vi "FPGA_ADSRFilter.vi"(11 "ADSR Settings":T1) -> ()   [LabVIEW 2014]
uses:
  Desktop/Envelope Filter/ADSR State.ctl
  <vilib>/rvi/FXPMathLib/FxpDiv/subVIs/nifxpmath_Div_SimConfig.ctl
  <vilib>/rvi/Emulation/niFpgaGetClockAttributes.vi
  <vilib>/rvi/Emulation/niFpgaSctlEmulationGetInTimedLoop.vi
  <vilib>/rvi/Emulation/niFpgaEmulationReportErrorSimple.vi
  <vilib>/rvi/FXPMathLib/FxpDiv/simVIs/DllFxpDivTemp_sub.vi
  <vilib>/rvi/Emulation/niFpgaCriticalErrorInLSC.vi
  MIDI/Controls/Stop.vi
  <vilib>/rvi/FXPMathLib/FxpDiv/XNode/nifxpmath_Div.xnode
  <vilib>/rvi/FXPMathLib/FxpMul/XNode/nifxpmath_Multiplier.xnode
  <vilib>/rvi/FXPMathLib/FxpSub/XNode/nifxpmath_Sub.xnode
  <vilib>/rvi/FXPMathLib/sim/FxpSim.dll
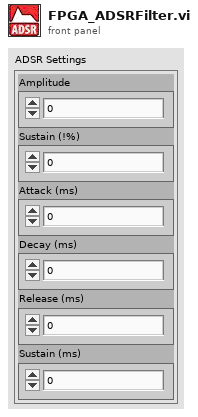
[diagram p1: front panel]
types:
  T1 = cluster{"Amplitude":fxp<+,10,1>, "Sustain (!%) ":fxp<+,10,1>, "Attack (ms)":fxp<+,11,11>, "Decay (ms) ":fxp<+,11,11>, "Release (ms)":fxp<+,11,11>, "Sustain (ms)":fxp<+,11,11>}
  T2 = typedef "ADSR State.ctl" = enum16{"Attack", "Decay", "Sustain", "Release"}
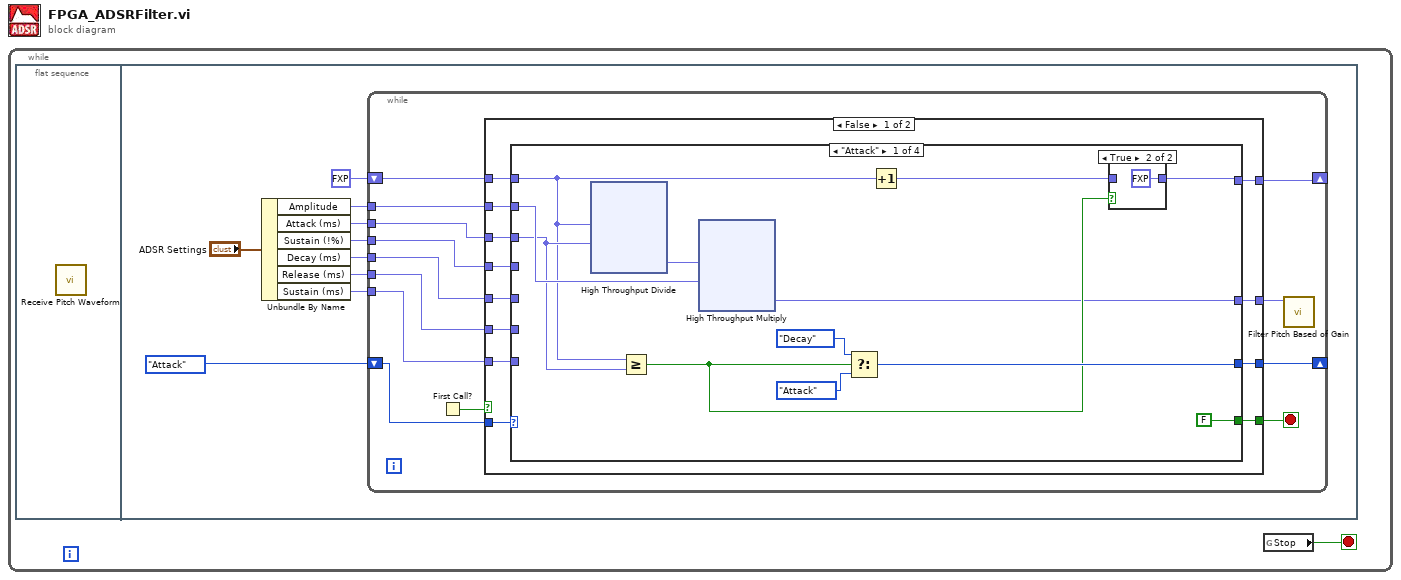
[diagram p0: block diagram]
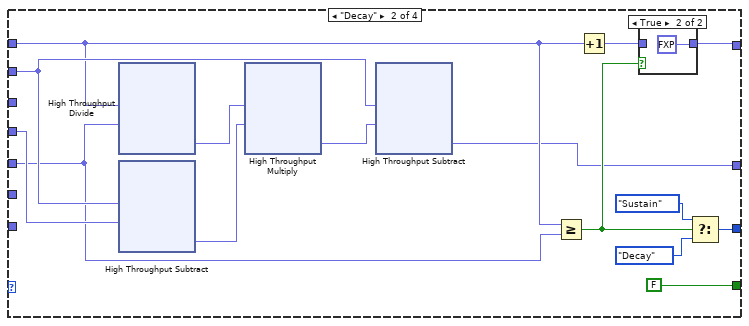
[diagram p3: hidden frame]
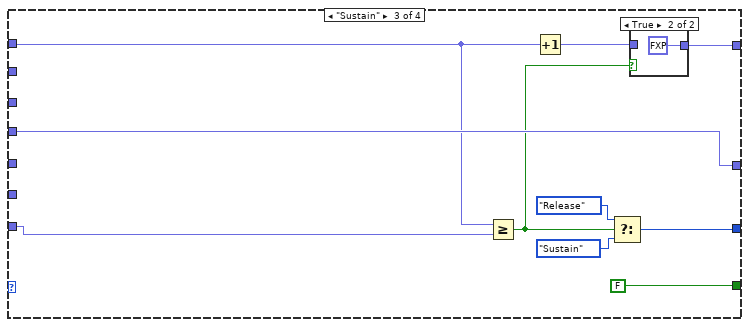
[diagram p5: hidden frame]
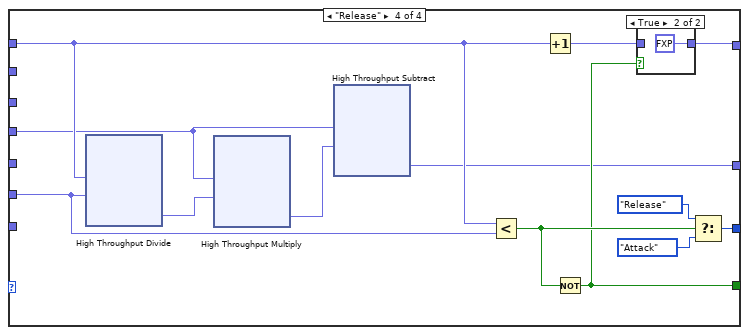
[diagram p7: hidden frame]
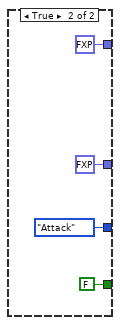
[diagram p9: hidden frame]
diagram:
  n1 = while {
    stop <- w1 stop-if-true
    n2 = flat-sequence {
      frame #0 {
        n3 = call "Receive Pitch Waveform.vi"() -> ()  [unwired: 12 in]
      }
      frame #1 {
        n4 = Unbundle By Name("ADSR Settings") -> ("Amplitude"=w7:fxp<+,10,1>, "Attack (ms)"=w6:fxp<+,11,11>, "Sustain (!%)"=w5:fxp<+,10,1>, "Decay (ms)"=w4:fxp<+,11,11>, "Release (ms)"=w3:fxp<+,11,11>, "Sustain (ms)"=w2:fxp<+,11,11>)
        n5 = while {
          shift-right: [w22] -> _
          shift-left: ADSR_State."Attack" -> [w23]
          shift-right: [w20] -> _
          shift-left: fxp<+,11,11> 0.0 ("Amplitude") -> [w19]
          tunnel: w7 -> [w16]
          tunnel: w6 -> [w15]
          tunnel: w5 -> [w14]
          tunnel: w4 -> [w13]
          tunnel: w3 -> [w12]
          tunnel: w2 -> [w11]
          stop <- w21 stop-if-true
          n6 = First Call?() -> (First Call?: T/F=w18:bool)
          n7 = case shown="False" w18 {
            tunnel: w23 -> [w35 _]
            tunnel: [w34 ADSR_State."Attack"] -> w22
            tunnel: [w33 FALSE] -> w21
            tunnel: [w32 fxp<+,10,1> 0.0 ("x-y")] -> w17
            tunnel: [w31 fxp<+,11,11> 0.0 ("Amplitude")] -> w20
            tunnel: w19 -> [w30 _]
            tunnel: w11 -> [w29 _]
            tunnel: w12 -> [w28 _]
            tunnel: w13 -> [w27 _]
            tunnel: w14 -> [w26 _]
            tunnel: w15 -> [w25 _]
            tunnel: w16 -> [w24 _]
            frame False {
              n8 = case shown="\"Attack\"" w35 {
                tunnel: w30 -> [w41 w81 w124 w140]
                tunnel: w24 -> [w46 w88 _ _]
                tunnel: w26 -> [_ w91 w126 w133]
                tunnel: w25 -> [w45 _ _ _]
                tunnel: w27 -> [_ w80 _ _]
                tunnel: w28 -> [_ _ _ w137]
                tunnel: [w42 w84 w127 w143] -> w34
                tunnel: [FALSE FALSE FALSE w136] -> w33
                tunnel: [w37 w78 w126 w135] -> w32
                tunnel: w29 -> [_ _ w122 _]
                tunnel: [w36 w77 w123 w134] -> w31
                frame "Attack" {
                  n9 = xnode "High Throughput Divide"("x"=w41, "y"=w45) -> ("x/y"=w47:fxp<+,10,1>)
                  n10 = Greater Or Equal?(x=w41, y=w45) -> (x >= y?=w39:bool)
                  n11 = xnode ("High Throughput Multiply")("x"=w47, "y"=w46) -> ("x*y"=w37:fxp<+,10,1>)
                  n12 = Select(t=ADSR_State."Decay", s=w39, f=ADSR_State."Attack") -> (s? t:f=w42:T2)
                  n13 = Increment(x=w41) -> (x+1=w38:fxp<+,11,11>)
                  n14 = case shown="True" w39 {
                    tunnel: w38 -> [w48 _]
                    tunnel: [w48 fxp<+,11,11> 0.0 ("Amplitude")] -> w36
                    frame False {
                    }
                    frame True {
                    }
                  }
                }
                frame "Decay" {
                  n15 = xnode "High Throughput Divide"("x"=w81, "y"=w80) -> ("x/y"=w90:fxp<+,10,1>)
                  n16 = xnode "High Throughput Subtract"("x"=w88, "y"=w91) -> ("x-y"=w89:fxp<+,10,1>)
                  n17 = xnode ("High Throughput Multiply")("x"=w90, "y"=w89) -> ("x*y"=w79:fxp<+,10,1>)
                  n18 = xnode "High Throughput Subtract"("x"=w88, "y"=w79) -> ("x-y"=w78:fxp<+,10,1>)
                  n19 = Greater Or Equal?(x=w81, y=w80) -> (x >= y?=w82:bool)
                  n20 = Increment(x=w81) -> (x+1=w83:fxp<+,11,11>)
                  n21 = case shown="True" w82 {
                    tunnel: w83 -> [w92 _]
                    tunnel: [w92 fxp<+,11,11> 0.0 ("Amplitude")] -> w77
                    frame False {
                    }
                    frame True {
                    }
                  }
                  n22 = Select(t=ADSR_State."Sustain", s=w82, f=ADSR_State."Decay") -> (s? t:f=w84:T2)
                }
                frame "Sustain" {
                  n23 = Greater Or Equal?(x=w124, y=w122) -> (x >= y?=w121:bool)
                  n24 = Increment(x=w124) -> (x+1=w125:fxp<+,11,11>)
                  n25 = Select(t=ADSR_State."Release", s=w121, f=ADSR_State."Sustain") -> (s? t:f=w127:T2)
                  n26 = case shown="True" w121 {
                    tunnel: [w131 fxp<+,11,11> 0.0 ("Amplitude")] -> w123
                    tunnel: w125 -> [w131 _]
                    frame False {
                    }
                    frame True {
                    }
                  }
                }
                frame "Release" {
                  n27 = xnode "High Throughput Divide"("x"=w140, "y"=w137) -> ("x/y"=w142:fxp<+,10,1>)
                  n28 = xnode ("High Throughput Multiply")("x"=w133, "y"=w142) -> ("x*y"=w141:fxp<+,10,1>)
                  n29 = xnode "High Throughput Subtract"("x"=w133, "y"=w141) -> ("x-y"=w135:fxp<+,10,1>)
                  n30 = Less?(x=w140, y=w137) -> (x < y?=w139:bool)
                  n31 = Increment(x=w140) -> (x+1=w138:fxp<+,11,11>)
                  n32 = Not(x=w139) -> (.not. x?=w136:bool)
                  n33 = case shown="True" w136 {
                    tunnel: w138 -> [w146 _]
                    tunnel: [w146 fxp<+,11,11> 0.0 ("Amplitude")] -> w134
                    frame False {
                    }
                    frame True {
                    }
                  }
                  n34 = Select(t=ADSR_State."Release", s=w139, f=ADSR_State."Attack") -> (s? t:f=w143:T2)
                }
              }
            }
            frame True {
            }
          }
          n35 = call "Filter Pitch Based of Gain.vi"("Gain"=w17) -> ()  [unwired: 11 in]
        }
      }
    }
    n36 = global read "Stop.vi" "Stop"() -> (w1:bool)
  }
